vi "save_bin.vi"(4 "SigArray":waveform(i16)[](array[waveform]), 5 "DevNo":i32, 6 "timestamp":timestamp, 7 "start path":path) -> (0 "error out":errorcluster, 3 "final Path":path)   [LabVIEW 2010]
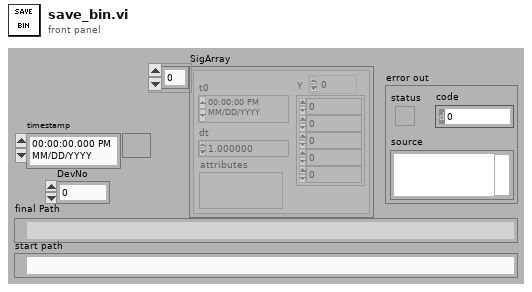
[diagram p1: front panel]
types:
  T1 = enum16{"open", "open or create", "create or replace", "create", "open (read-only)"}
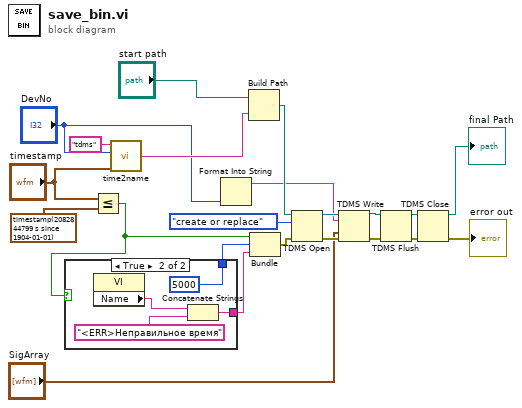
[diagram p0: block diagram]
diagram:
  n1 = Less Or Equal?(x="timestamp", y=timestamp(2082844799 s since 1904-01-01) ("timestamp")) -> (x <= y?=w1:bool)
  n2 = case shown="True" w1 {
    tunnel: [_ 5000] -> w3
    tunnel: [_ w23] -> w2
    frame False {
    }
    frame True {
      n3 = property class="VI"() -> ("Name"=w25:string)  [unwired: 2 in, 2 out]
      n4 = Concatenate Strings(w25, "<ERR>Неправильное время" ("string")) -> (w23:string)
    }
  }
  n5 = call "time2name.vi"("timestamp"="timestamp", "DevNo"="DevNo", "ext"="tdms") -> ("String"=w22:string)  [unwired: 1 in]
  n6 = Format Into String("DevNo") -> (resulting string=w12:string)  [unwired: 3 in, 1 out]
  n7 = Build Path(base path="start path", name or relative path=w22) -> (appended path=w16:path)
  n8 = Bundle(w1, w3, w2) -> (w6:errorcluster)  [unwired: 1 in]
  n9 = TDMS Open(8:w6, 10:T1."create or replace" ("operation (0:open)"), 11:w16) -> (0:w20:errorcluster, 3:w19:refnum<k34>)  [unwired: 3 in]
  n10 = TDMS Write(0:w19, 5:w12, 9:"SigArray", 11:w20) -> (4:w11:refnum<k34>, 15:w10:errorcluster)  [unwired: 2 in, 2 out]
  n11 = TDMS Flush(4:w10, 7:w11) -> (0:w8:errorcluster, 3:w9:refnum<k34>)
  n12 = TDMS Close(8:w8, 11:w9) -> (0:→"error out":errorcluster, 3:→"final Path":path)
